vi "Utility Clean Up Initialize.vi"(0 "VISA session":refnum<visa-resource-name>, 11 "error in (no error)":errorcluster) -> (4 "dup VISA session":refnum<visa-resource-name>, 15 "error out":errorcluster)   [LabVIEW 2019, in "Lake Shore Cryotronics 331.lvlib"]
doc: "This Utility VI closes any open VISA sessions in the event that there is an error during an initialization. It is called only from the LSCI 331 Initialize VI, and is not meant to be altered. Changing this VI can cause the LSCI 331 Initialize VI to operate improperly."
uses:
  <instrlib>/Lake Shore Cryotronics 331/Lake Shore Cryotronics 331.lvlib
panel:
  in  "VISA session (for class)":refnum<visa-resource-name>
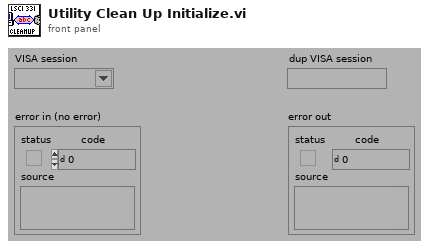
[diagram p1: front panel]
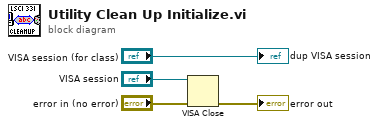
[diagram p0: block diagram]
diagram:
  n1 = VISA Close(VISA resource name="VISA session", error in (no error)="error in (no error)") -> (error out=→"error out":errorcluster)
  "dup VISA session" <- "VISA session (for class)"
